vi "PWM FPGA test.vi"() -> ()   [LabVIEW 2012]
uses:
  <vilib>/Platform/TimedLoop/XDataNode/timing_clust.ctl
  <vilib>/Platform/TimedLoop/XDataNode/nitl_modes.ctl
  <vilib>/Platform/TimedLoop/XDataNode/wakeup.ctl
  <vilib>/rvi/Emulation/niFpgaSctlEmulationRegisterWithScheduler.vi
  <vilib>/rvi/eio/common/nirviEmuTemplateMethod_errors.vi
  <vilib>/rvi/Emulation/niFpgaSctlEmulationScheduler.vi
  <vilib>/Platform/TimedLoop/XDataNode/XDataNode.xnode
  <vilib>/eio/EIONode/EIONode.xnode
  <vilib>/Platform/TimedLoop/XDataNode/XDNodeRunTimeDep.lvlib
panel:
  in  "TTL 1":bool
  in  "TTL 0":bool
  in  "ISO Out 2":bool
  in  "ISO Out 1":bool
  in  "ISO Out 0":bool
  in  "frequency (periods/tick)":fxp<+,32,0>=0.0007812499534338713
  in  "duty cycle (periods)":fxp<+,16,0>=0.5
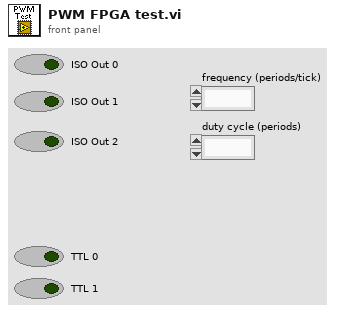
[diagram p1: front panel]
types:
  T1 = typedef "XDNodeRunTimeDep.lvlib/timing_clust.ctl" = cluster{"Expected End [f-1]":u64, "Actual End [f-1]":u64, "Finished Late? [f-1]":bool, "Expected End [i-1]":u64, "Actual End [i-1]":u64, "Finished Late? [i-1]":bool, "Expected Start [i]":u64, "Actual Start [i]":u64, "Expected Start [f]":u64, "Actual Start [f]":u64, "Source Name":string, "Structure Name":string, "Period":i64, "Deadline":i64, "Offset":i64, "Start":i64, "Priority":i32, "Timeout":i32, "Mode":T2, "Wakeup Reason":T3, "Error":errorcluster, "Source Type":string, "Secondary Source Type":string, "Global End Time":u64, "Global Start Time":u64, "Frame Duration":u64, "Iteration Duration":u64, "Assigned CPU":i32, "I/O Scan Engine Mode":u32}
  T2 = typedef "XDNodeRunTimeDep.lvlib/nitl_modes.ctl" = enum32{"No Change", "Process missed periods, maintain original phase", "Discard missed periods, maintain original phase", "Process missed periods, ignore original phase", "Discard missed periods, ignore original phase"}
  T3 = typedef "XDNodeRunTimeDep.lvlib/wakeup.ctl" = enum32{"Normal", "Aborted", "Asynchronous wakeup", "Timing source error", "Timed loop error", "Timeout"}
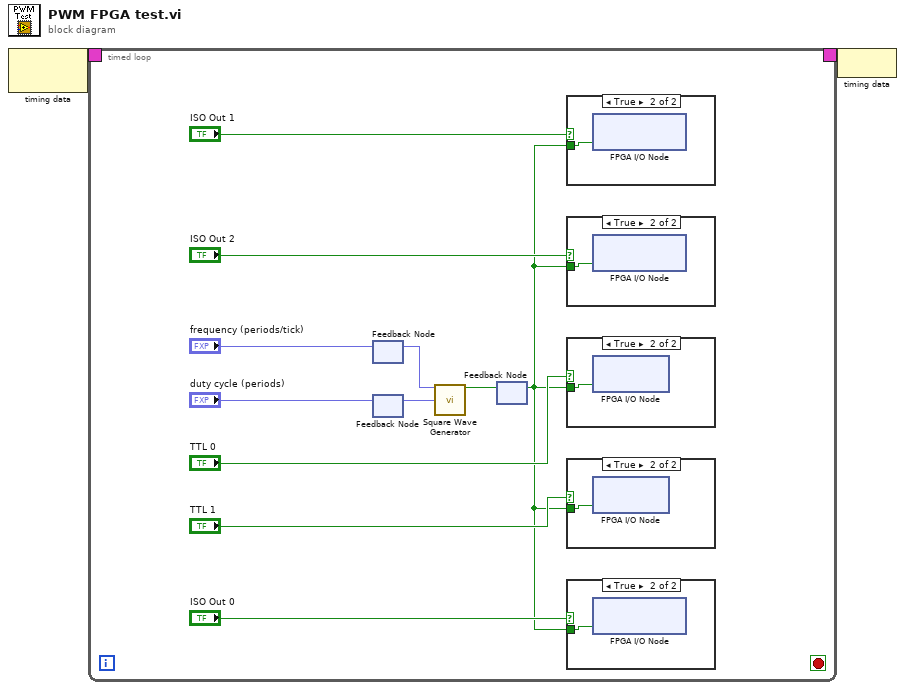
[diagram p0: block diagram]
diagram:
  n1 = node-c288() -> (w2:T1)  [unwired: 1 in]
  n2 = timed-loop {
    timing: w2 -> [_]
    timing-out: [_] -> w1
    stop <- _ stop-if-true
    n3 = feedback-in #1("frequency (periods/tick)") -> ()
    n4 = feedback #1() -> (w10:fxp<+,32,0>)  [unwired: 1 in]
    n5 = feedback-in #2("duty cycle (periods)") -> ()
    n6 = feedback #2() -> (w9:fxp<+,16,0>)  [unwired: 1 in]
    n7 = call "Square Wave Generator"("frequency (periods/tick)"=w10, "duty cycle (periods)"=w9) -> ("square wave out"=w11:bool)  [unwired: 13 in]
    n8 = feedback-in #3(w11) -> ()
    n9 = feedback #3() -> (w3:bool)  [unwired: 1 in]
    n10 = case shown="True" "ISO Out 1" {
      tunnel: w3 -> [_ w17]
      frame False {
      }
      frame True {
        n11 = xnode "FPGA I/O Node"("ISO Out 1"=w17) -> ()  [unwired: 1 in, 1 out]
      }
    }
    n12 = case shown="True" "ISO Out 2" {
      tunnel: w3 -> [_ w16]
      frame False {
      }
      frame True {
        n13 = xnode "FPGA I/O Node"("ISO Out 2"=w16) -> ()  [unwired: 1 in, 1 out]
      }
    }
    n14 = case shown="True" "TTL 0" {
      tunnel: w3 -> [_ w15]
      frame False {
      }
      frame True {
        n15 = xnode "FPGA I/O Node"("TTL 0"=w15) -> ()  [unwired: 1 in, 1 out]
      }
    }
    n16 = case shown="True" "TTL 1" {
      tunnel: w3 -> [_ w14]
      frame False {
      }
      frame True {
        n17 = xnode "FPGA I/O Node"("TTL 1"=w14) -> ()  [unwired: 1 in, 1 out]
      }
    }
    n18 = case shown="True" "ISO Out 0" {
      tunnel: w3 -> [_ w18]
      frame False {
      }
      frame True {
        n19 = xnode "FPGA I/O Node"("ISO Out 0"=w18) -> ()  [unwired: 1 in, 1 out]
      }
    }
  }
  n20 = node-c288(w1) -> ()
